vi "CU_SaveSubset.vi"(8 "CLassLabels":string[](array[string]), 9 "EEG Feature Vectors":T1[](array[typedef]), 10 "Suffix":string, 11 "XML file path":path) -> (0 "error out":errorcluster)   [LabVIEW 2016, in "Classifier.lvlib"]
uses:
  _XML_EEG_Features/XML_FF_Trial.ctl
  _XML_EEG_Features/XML_FF_Header.ctl
  <vilib>/xml/Close Reference(Node).vi
  Classifier.lvlib
  _XML_EEG_Features/XML_EEG_Features.lvlib
  <vilib>/xml/NI_XML.lvlib
panel:
  # "This VI is a part of BCI Design library, http://www.ru-bci.org \nCopyright © 2020, Sotnikov Peter, All rights reserved. License: GNU GPLv3"
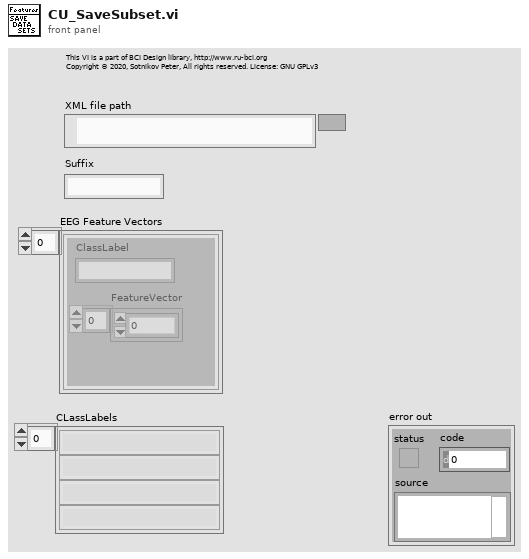
[diagram p1: front panel]
types:
  T1 = typedef "XML_EEG_Features.lvlib/XML_FF_Trial.ctl" = cluster{"ClassLabel":string, "FeatureVector":dbl[]}
  T2 = typedef "XML_EEG_Features.lvlib/XML_FF_Header.ctl" = cluster{"NumberOfTrials":i32, "NumberOfClasses":i32, "FeatureVectorLength":i32, "FeatureExtractionMethod":string}
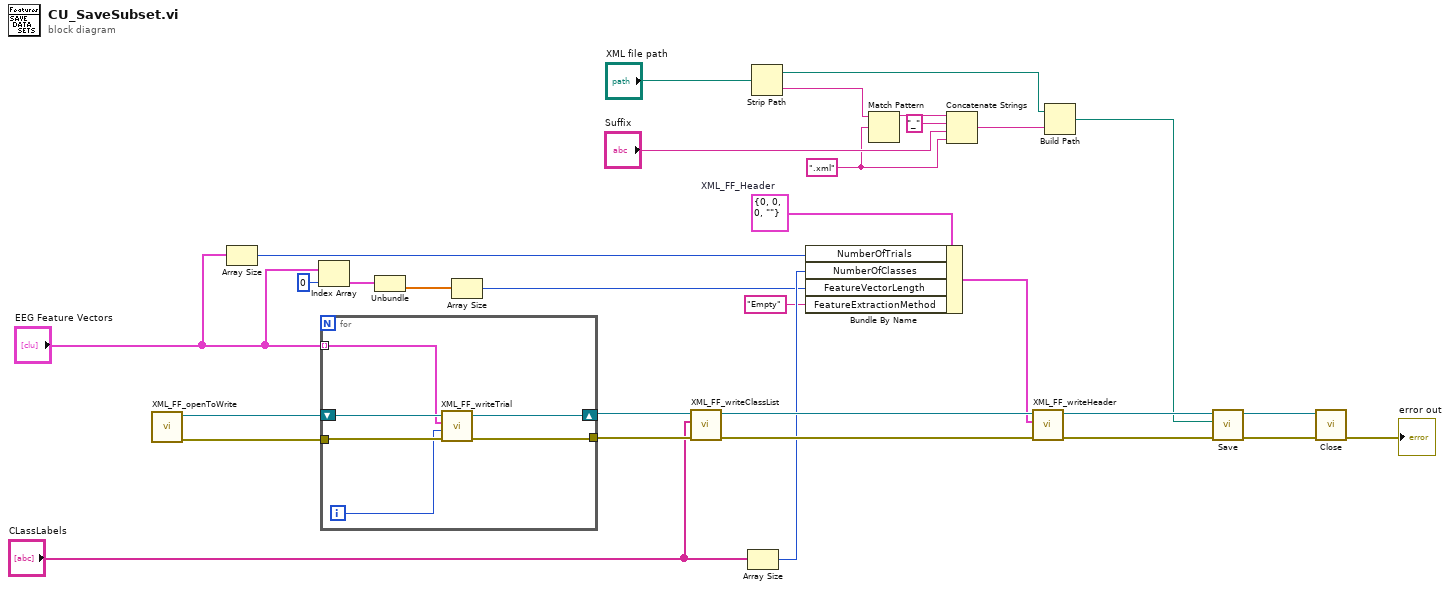
[diagram p0: block diagram]
diagram:
  w6 = ".xml" ("regular expression")
  w24 = T2 {"NumberOfTrials"=0, "NumberOfClasses"=0, "FeatureVectorLength"=0, "FeatureExtractionMethod"=""}  # XML_FF_Header
  n1 = call "XML_FF_openToWrite.vi"() -> ("error out"=w30:errorcluster, "DOM document out"=w31:refnum<k20>)  [unwired: 10 in]
  n2 = Array Size(array="EEG Feature Vectors") -> (size(s)=w23:i32)
  n3 = Index Array(array="EEG Feature Vectors", index=0) -> (element=w20:T1)
  n4 = for {
    shift-right: [w35] -> w29
    shift-left: w31 -> [w37]
    tunnel: w30 -> [w36]
    tunnel: "EEG Feature Vectors" -> [w34] mode=indexing
    tunnel: [w32] -> w28
    i -> [w33]
    n5 = call "XML_FF_writeTrial.vi"("error in (no error)"=w36, "Trial Number"=w33, "XML_FF_Trial"=w34, "DOM document in"=w37) -> ("error out"=w32:errorcluster, "DOM document out"=w35:refnum<k20>)  [unwired: 6 in]
  }
  n6 = Unbundle(w20) -> ("FeatureVector"=w19:dbl[])  [unwired: 1 out]
  n7 = Array Size(array=w19) -> (size(s)=w18:i32)
  n8 = call "XML_FF_writeClassList.vi"("error in (no error)"=w28, "ClassList"="CLassLabels", "DOM document in"=w29) -> ("error out"=w25:errorcluster, "DOM document out"=w26:refnum<k20>)  [unwired: 7 in]
  n9 = Array Size(array="CLassLabels") -> (size(s)=w22:i32)
  n10 = Strip Path(path="XML file path") -> (stripped path=w4:path, name=w9:string)
  n11 = Bundle By Name(cluster=w24, "NumberOfTrials"=w23, "NumberOfClasses"=w22, "FeatureVectorLength"=w18, "FeatureExtractionMethod"="Empty") -> (w16:T2)
  n12 = Match Pattern(string=w9, regular expression=w6) -> (before substring=w8:string)  [unwired: 1 in, 3 out]
  n13 = Concatenate Strings(w8, "_" ("string"), "Suffix", w6) -> (w3:string)
  n14 = call "XML_FF_writeHeader.vi"("error in (no error)"=w25, "XML_FF_Header"=w16, "DOM document in"=w26) -> ("error out"=w14:errorcluster, "DOM document out"=w15:refnum<k20>)  [unwired: 7 in]
  n15 = Build Path(base path=w4, name or relative path=w3) -> (appended path=w2:path)
  n16 = call <vilib>:"Save.vi"("error in (no error)"=w14, "XML file path"=w2, "DOM document in"=w15) -> ("error out"=w12:errorcluster, "DOM document out"=w13:refnum<k20>)  [unwired: 6 in, 1 out]
  n17 = call-poly <vilib>:"Close.vi"("error in (no error)"=w12, "node"=w13) -> ("error out"=→"error out":errorcluster)  [unwired: 7 in]
